vi "list_documents.vi"(8 "error in":errorcluster, 11 "Device In":T1) -> (0 "error out":errorcluster, 3 "Device Out":T1)   [LabVIEW 2019]
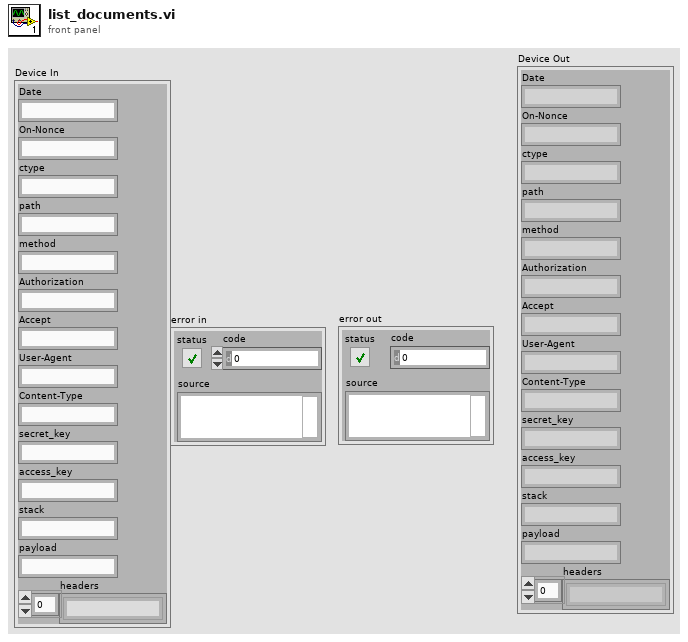
[diagram p1: front panel]
types:
  T1 = cluster{"Date":string, "On-Nonce":string, "ctype":string, "path":string, "method":string, "Authorization":string, "Accept":string, "User-Agent":string, "Content-Type":string, "secret_key":string, "access_key":string, "stack":string, "payload":string, "headers":string[]}
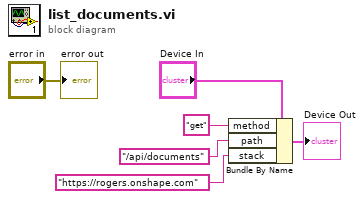
[diagram p0: block diagram]
diagram:
  n1 = Bundle By Name(cluster="Device In", "method"="get" ("Method"), "path"="/api/documents" ("payload"), "stack"="https://rogers.onshape.com" ("stacks")) -> (→"Device Out":T1)
  "error out" <- "error in"
